vi "SngJntArmSim_EstimateMOI.vi"(9 "ArmMass_Kg":dbl=1.0, 11 "ArmLength_M":dbl=1.0) -> (3 "MOI":dbl)   [LabVIEW 2019, in "Trajectory_Library.lvlib"]
doc: "Creates a new LINEAR SYSTEM data cluster with the specified values. \n\n\nInputs: \n - XXX -- XXX.\n\nOutputs:\n - XXX -- XXX."
uses:
  Trajectory_Library.lvlib
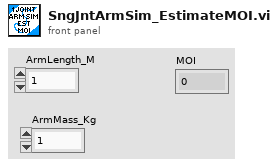
[diagram p1: front panel]
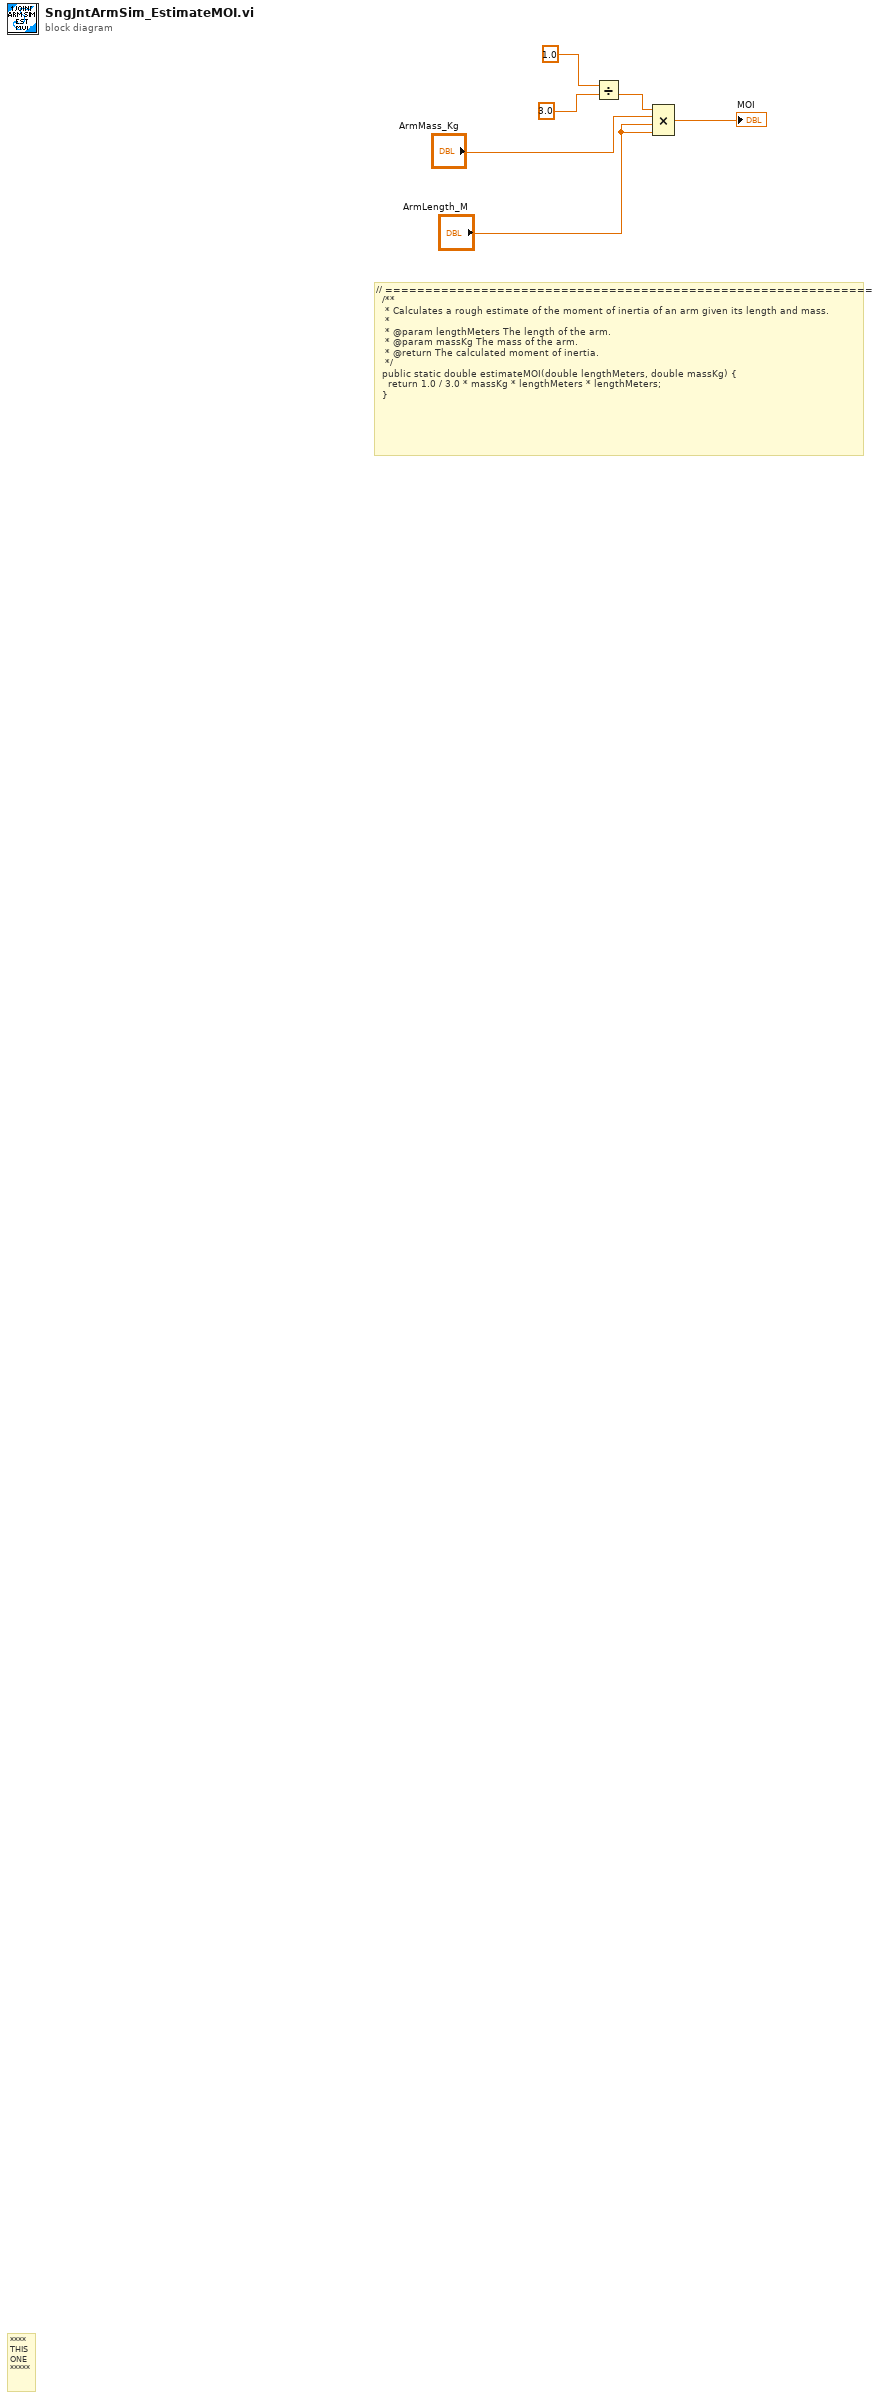
[diagram p0: block diagram]
diagram:
  # "// ==============================================================\n  /**\n   * Calculates a rough estimate of the moment of inertia of an arm given its length and mass.\n   *\n   * @param lengthMeters The length of the arm.\n   * @param massKg The mass of the arm.\n   * @return The calculated moment of inertia.\n   */\n  public static double estimateMOI(double lengthMeters, double massKg) {\n    return 1.0 / 3.0 * massKg * lengthMeters * lengthMeters;\n  }"
  # "****\nTHIS\nONE\n*****"
  n1 = Divide(x=1.0, y=3.0) -> (x/y=w4:dbl)
  n2 = Compound Arithmetic op=MULTIPLY(w4, "ArmMass_Kg", "ArmLength_M", "ArmLength_M") -> (→"MOI":dbl)
